vi "Stop All.vi"(8 "error in":errorcluster, 10 "stop configuration (all)":T1={"Stop the monitor? (true)"=TRUE, "Stop the remote terminals? (true)"=TRUE, "Stop the bus controller? (true)"=TRUE}, 11 "module reference":T2) -> (0 "error out":errorcluster {"code" format="%x"}, 3 "module reference out":T2)   [LabVIEW 2020, in "AIM MIL-STD-1553 Hardware API.lvlib"]
uses:
  AIM MIL-STD-1553 Hardware API.lvlib
  Module Reference.ctl
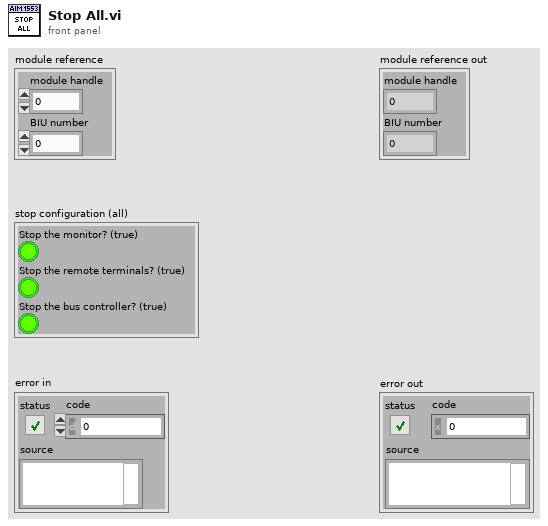
[diagram p1: front panel]
types:
  T1 = cluster{"Stop the monitor? (true)":bool, "Stop the remote terminals? (true)":bool, "Stop the bus controller? (true)":bool}
  T2 = typedef "AIM MIL-STD-1553 Hardware API.lvlib/Module Reference.ctl" = cluster{"module handle":u32, "BIU number":u8}
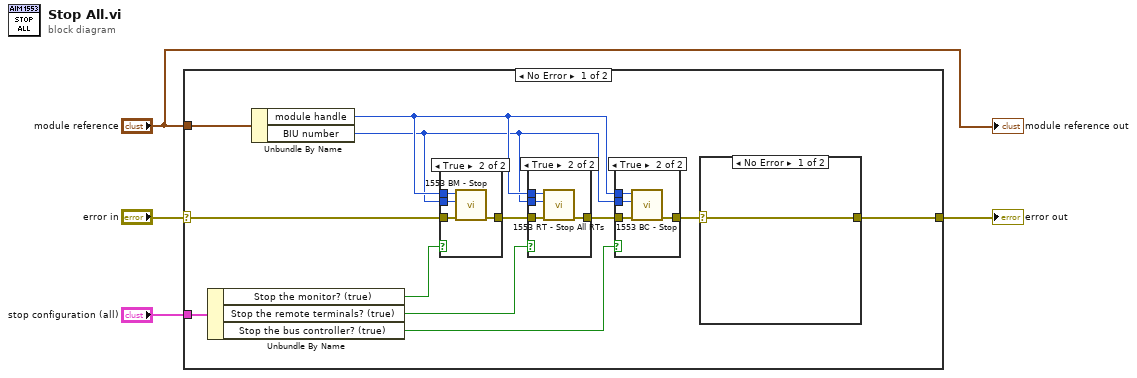
[diagram p0: block diagram]
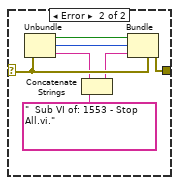
[diagram p3: hidden frame]
diagram:
  n1 = case shown="No Error" "error in" {
    selector: "error in" -> [w10 w40]
    tunnel: [w5 w40] -> w4
    tunnel: "module reference" -> [w13 _]
    tunnel: "stop configuration (all)" -> [w9 _]
    frame No Error {
      n2 = Unbundle By Name(w9) -> ("Stop the monitor? (true)"=w8:bool, "Stop the remote terminals? (true)"=w7:bool, "Stop the bus controller? (true)"=w6:bool)
      n3 = Unbundle By Name(w13) -> ("module handle"=w12:u32, "BIU number"=w11:u8)
      n4 = case shown="True" w8 {
        tunnel: w10 -> [w35 w39]
        tunnel: [w35 w38] -> w14
        tunnel: w11 -> [_ w37]
        tunnel: w12 -> [_ w36]
        frame False {
        }
        frame True {
          n5 = call <instrlib>:"1553 BM - Stop.vi"("Error In (none)"=w39, "BIU Number (1)"=w37, "Module Handle"=w36) -> ("Error Out"=w38:errorcluster)  [unwired: 8 in]
        }
      }
      n6 = case shown="True" w7 {
        tunnel: w14 -> [w30 w34]
        tunnel: [w30 w33] -> w15
        tunnel: w11 -> [_ w32]
        tunnel: w12 -> [_ w31]
        frame False {
        }
        frame True {
          n7 = call <instrlib>:"1553 RT - Stop All RTs.vi"("Error In (none)"=w34, "BIU Number (1)"=w32, "Module Handle"=w31) -> ("Error Out"=w33:errorcluster)  [unwired: 8 in]
        }
      }
      n8 = case shown="True" w6 {
        tunnel: w15 -> [w17 w21]
        tunnel: w11 -> [_ w20]
        tunnel: w12 -> [_ w19]
        tunnel: [w17 w18] -> w16
        frame False {
        }
        frame True {
          n9 = call <instrlib>:"1553 BC - Stop.vi"("Error In (none)"=w21, "BIU Number (1)"=w20, "Module Handle"=w19) -> ("Error Out"=w18:errorcluster)  [unwired: 8 in]
        }
      }
      n10 = case shown="No Error" w16 {
        selector: w16 -> [w22 w29]
        tunnel: [w22 w26] -> w5
        frame No Error {
        }
        frame Error {
          n11 = Unbundle(w29) -> ("status"=w27:bool, "code"=w28:i32, "source"=w25:string)
          n12 = Concatenate Strings(w25, "  Sub VI of: 1553 - Stop All.vi.") -> (w24:string)
          n13 = Bundle(cluster=w29, "status"=w27, "code"=w28, "source"=w24) -> (w26:errorcluster)
        }
      }
    }
    frame Error {
    }
  }
  "error out" <- w4
  "module reference out" <- "module reference"
